vi "Clear All Discretes.vi"(8 "error in":errorcluster, 11 "6509 in":refnum<class "6509.lvclass">) -> (0 "error out":errorcluster, 3 "6509 out":refnum<class "6509.lvclass">)   [LabVIEW 2019, in "6509.lvlib" / "6509.lvclass"]
uses:
  Library/6509.lvclass
  Library/6509.lvclass/6509.ctl
  <vilib>/DAQmx/write.llb/DAQmx Write (Digital 1D U8 NChan 1Samp).vi
  <vilib>/DAQmx/miscellaneous.llb/DAQmx Fill In Error Info.vi
  builds/Instruments/DIG_IO.lvlibp/Library/DIG_IO.lvclass
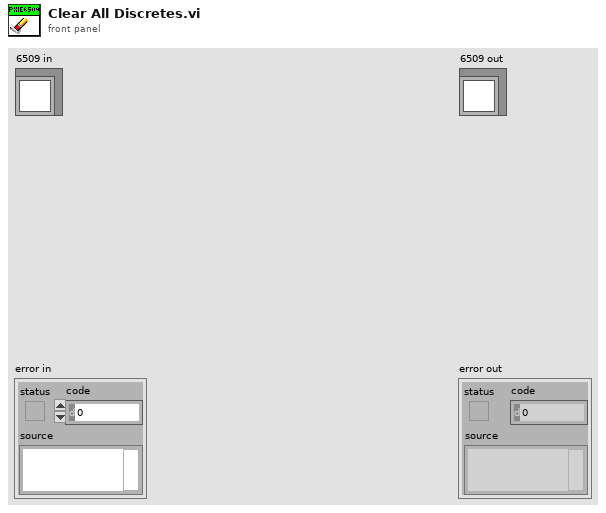
[diagram p1: front panel]
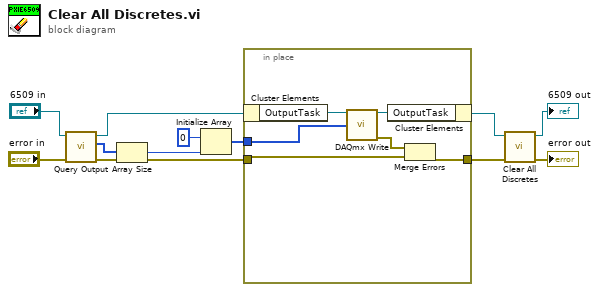
[diagram p0: block diagram]
diagram:
  n1 = call "Query Output.vi"("error in"="error in", "6509 in"="6509 in") -> ("error out"=w3:errorcluster, "Port Array"=w2:u8[], "6509 out"=w8:refnum<class "6509.lvclass">)  [unwired: 7 in]
  n2 = Array Size(array=w2) -> (size(s)=w1:i32)
  n3 = Initialize Array(u8 0, w1) -> (w5:u8[])
  n4 = in-place {
    in-place-border: w5 -> [w15]
    in-place-border: [w14] -> w4
    in-place-border: w3 -> [w13]
    n5 = in-place-cluster #1(w8) -> ("OutputTask"=w18:refnum<k21>)
    n6 = call-poly <vilib>:"DAQmx Write.vi"("task/channels in"=w18, "data"=w15) -> ("task out"=w17:refnum<k21>, "error out"=w16:errorcluster)  [unwired: 11 in, 1 out]
    n7 = in-place-cluster #1("OutputTask"=w17) -> (w10:refnum<class "6509.lvclass">)
    n8 = Merge Errors(w16, w13) -> (w14:errorcluster)
  }
  n9 = call-parent "Clear All Discretes.vi"("error in"=w4, "DIG_IO in"=w10) -> ("error out"=→"error out":errorcluster, "DIG_IO out"=→"6509 out":refnum<class "6509.lvclass">)  [unwired: 8 in]
